vi "Git_RepoInfo.vi"(4 "Your Password (not necessary)":string, 6 "Your User Name (not necessary)":string, 8 "error in (no error)":errorcluster, 10 "Repo Name":string, 11 "Repo User Name":string) -> (0 "error out":errorcluster, 1 "Not Found?":bool, 2 "body":string, 3 "headers":string="\n")   [LabVIEW 2012]
doc: "Gets the HEAD and BODY info for a given username/repo, and checks whether the repo exists."
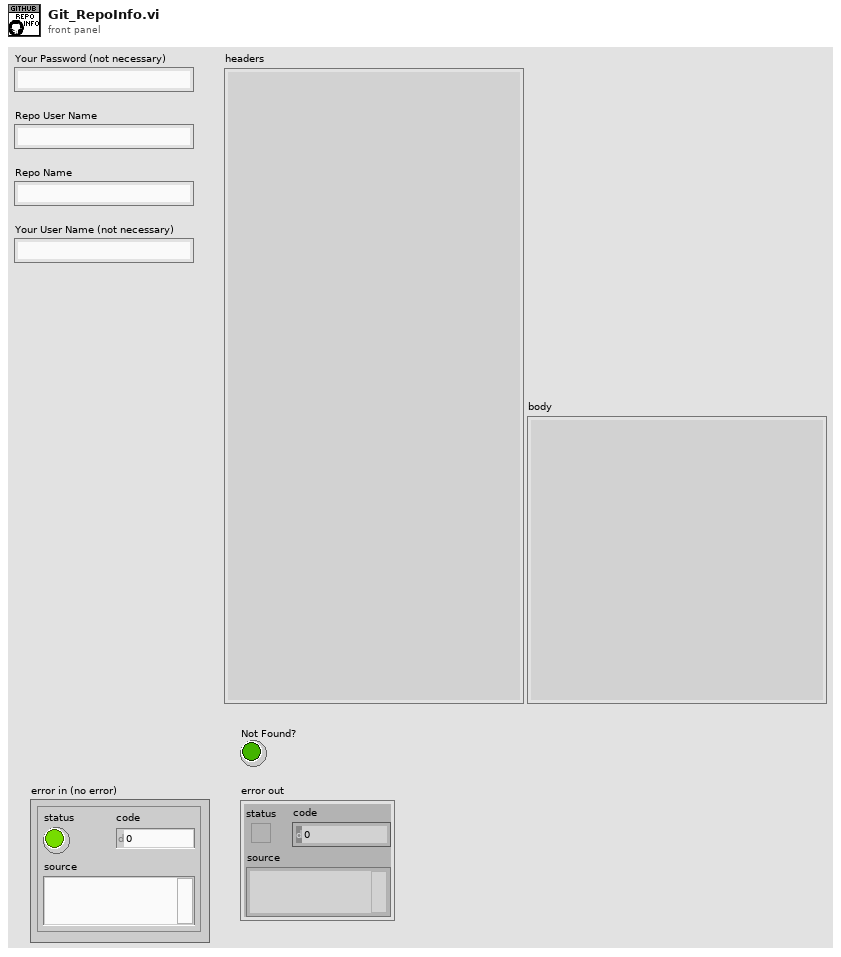
[diagram p1: front panel]
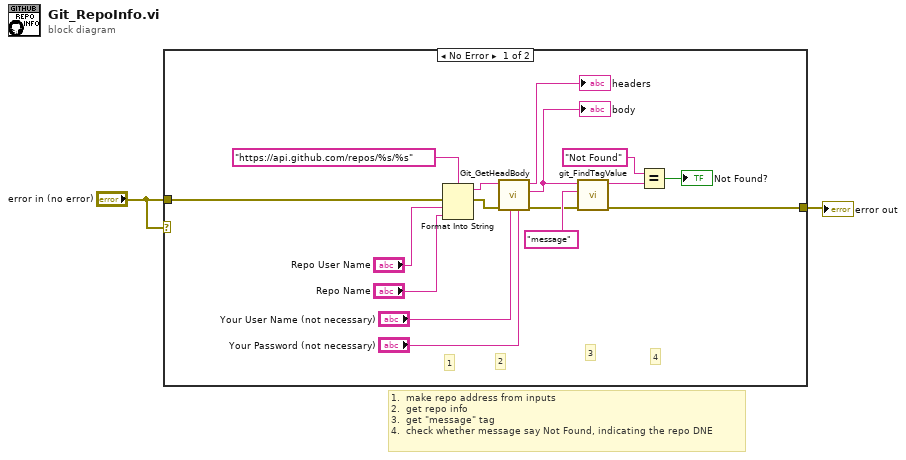
[diagram p0: block diagram]
diagram:
  # "1.  make repo address from inputs\n2.  get repo info\n3.  get \"message\" tag\n4.  check whether message say Not Found, indicating the repo DNE"
  n1 = case shown="No Error" "error in (no error)" {
    tunnel: [w18 w19] -> w2
    tunnel: "error in (no error)" -> [w11 w19]
    frame No Error {
      # "4"
      # "3"
      # "2"
      # "1"
      n2 = Format Into String(format string="https://api.github.com/repos/%s/%s", error in=w11, "Repo User Name", "Repo Name") -> (resulting string=w10:string, error out=w12:errorcluster)  [unwired: 1 in]
      n3 = call "Git_GetHeadBody.vi"("Your Password (not necessary)"="Your Password (not necessary)", "Your User Name (not necessary)"="Your User Name (not necessary)", "error in (no error)"=w12, "Address"=w10) -> ("error out"=w5:errorcluster, "body"=w13:string, "headers"=→"headers":string)  [unwired: 5 in]
      "body" <- w13
      n4 = call "git_FindTagValue.vi"("Error In"=w5, "Tag Name"="message", "Text"=w13) -> ("Error Out"=w18:errorcluster, "Value"=w15:string)  [unwired: 4 in, 3 out]
      n5 = Equal?(x="Not Found", y=w15) -> (x = y?=→"Not Found?":bool)
    }
    frame Error {
    }
  }
  "error out" <- w2
